vi "Write Active.vi"(7 "SPI CS":refnum<class "SPI CS.lvclass">, 8 "error in (no error)":errorcluster, 10 "Active":bool, 11 "Session In":refnum<class "Session.lvclass">) -> (0 "error out":errorcluster, 3 "Session Out":refnum<class "Session.lvclass">)   [LabVIEW 2020, in "CTI.lvlib" / "SPI CS.lvclass"]
uses:
  SPI CS.lvclass
  SPI CS.lvclass/SPI CS.ctl
  GPIO/GPIO.lvclass
  Session/Session.lvclass
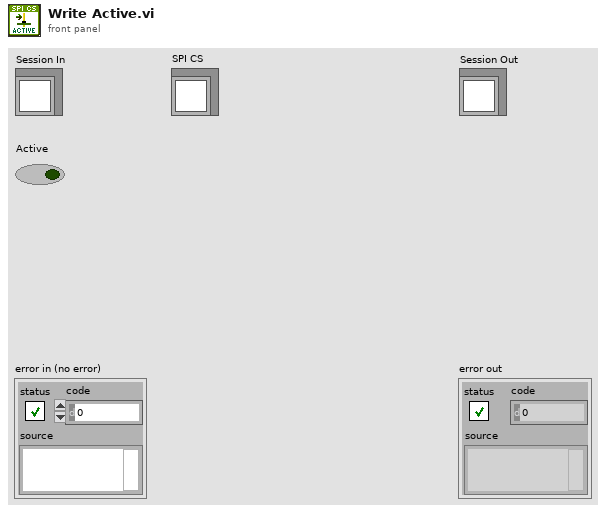
[diagram p1: front panel]
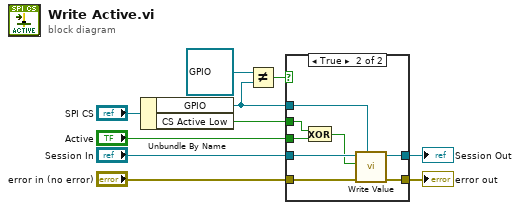
[diagram p0: block diagram]
diagram:
  n1 = Unbundle By Name("SPI CS") -> ("GPIO"=w3:refnum<class "GPIO.lvclass">, "CS Active Low"=w8:bool)
  n2 = Not Equal?(x=refnum<class "GPIO.lvclass"> refnum, y=w3) -> (x != y?=w1:bool)
  n3 = case shown="True" w1 {
    tunnel: "Active" -> [_ w20]
    tunnel: w8 -> [_ w19]
    tunnel: "Session In" -> [w12 w18]
    tunnel: "error in (no error)" -> [w11 w17]
    tunnel: [w11 w16] -> w5
    tunnel: [w12 w14] -> w4
    tunnel: w3 -> [_ w13]
    frame False {
    }
    frame True {
      n4 = Exclusive Or(1:w20, 2:w19) -> (0:w15:bool)
      n5 = call "Write Value.vi"("GPIO"=w13, "error in (no error)"=w17, "Value"=w15, "Session In"=w18) -> ("error out"=w16:errorcluster, "Session Out"=w14:refnum<class "Session.lvclass">)  [unwired: 6 in]
    }
  }
  "error out" <- w5
  "Session Out" <- w4
